vi "ZCAN_Resistance.vi"() -> ()   [LabVIEW 2018]
uses:
  bin/zlgcan_wrap.dll
panel:
  in  "enable":i32
  in  "can_index":u32
  in  "device_handle":u32
  out "set_Resistance_success?":bool
  out "error out":errorcluster caption="错误输出"
  in  "error in (no error)":errorcluster caption="错误输入（无错误）"
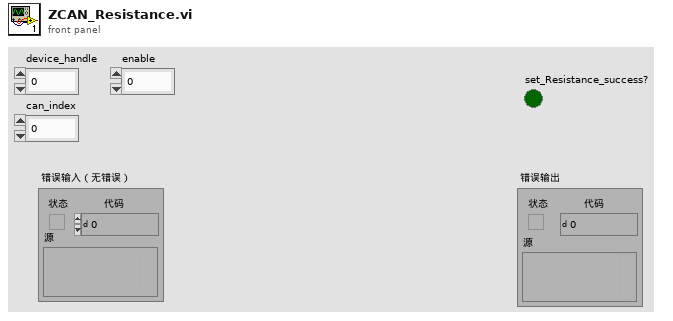
[diagram p1: front panel]
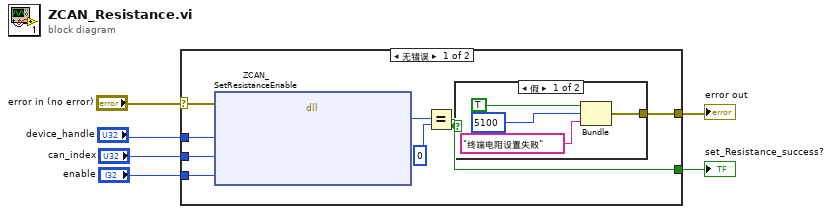
[diagram p0: block diagram]
diagram:
  n1 = case shown="无错误" "error in (no error)" {
    selector: "error in (no error)" -> [w10 w19]
    tunnel: [w13 w19] -> w5
    tunnel: [w11 _] -> w4
    tunnel: "device_handle" -> [w9 _]
    tunnel: "can_index" -> [w8 _]
    tunnel: "enable" -> [w7 _]
    frame No Error {
      n2 = dll-call lib="D:/USBCANFD DEMO/zlgcan_wrap_20191223/bin/zlgcan_wrap.dll" fn="ZCAN_SetResistanceEnable" ("ZCAN_StartCAN")(error in=w10, "device_handle"=w9, "can_index"=w8, "enable"=w7) -> ("return"=w12:u32)  [unwired: 5 in, 2 out]
      n3 = Equal?(x=w12, y=0) -> (x = y?=w11:bool)
      n4 = case shown="假" w11 {
        tunnel: [w15 _] -> w13
        frame False {
          n5 = Bundle("status"=TRUE, "code"=5100, "消息"="终端电阻设置失败") -> (w15:cluster{"status":bool, "code":i32, "消息":string})  [unwired: 1 in]
        }
        frame True {
        }
      }
    }
    frame Error {
    }
  }
  "error out" <- w5
  "set_Resistance_success?" <- w4
